vi "UpdateStatus.vi"(8 "error in (no error)":errorcluster, 10 "status":string, 11 "Interface in":refnum<class "Interface.lvclass">) -> (0 "error out":errorcluster, 3 "Interface out":refnum<class "Interface.lvclass">)   [LabVIEW 2018, in "Interface.lvclass"]
uses:
  Interface.lvclass
  Interface.lvclass/Interface.ctl
panel:
  in  "Camera Status":T1
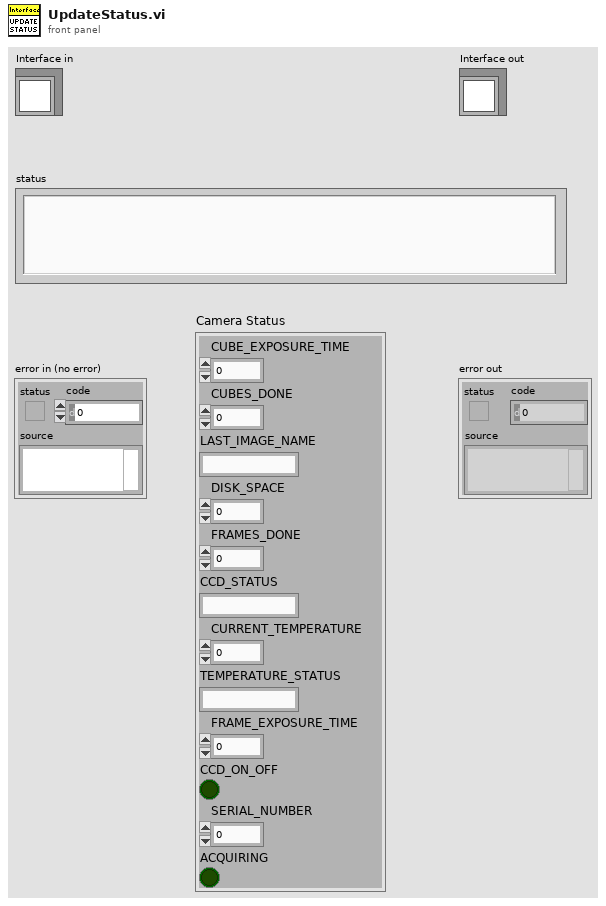
[diagram p1: front panel]
types:
  T1 = cluster{"CUBE_EXPOSURE_TIME":sgl, "CUBES_DONE":u16, "LAST_IMAGE_NAME":string, "DISK_SPACE":u16, "FRAMES_DONE":u16, "CCD_STATUS":string, "CURRENT_TEMPERATURE":i16, "TEMPERATURE_STATUS":string, "FRAME_EXPOSURE_TIME":u16, "CCD_ON_OFF":bool, "SERIAL_NUMBER":u16, "ACQUIRING":bool}
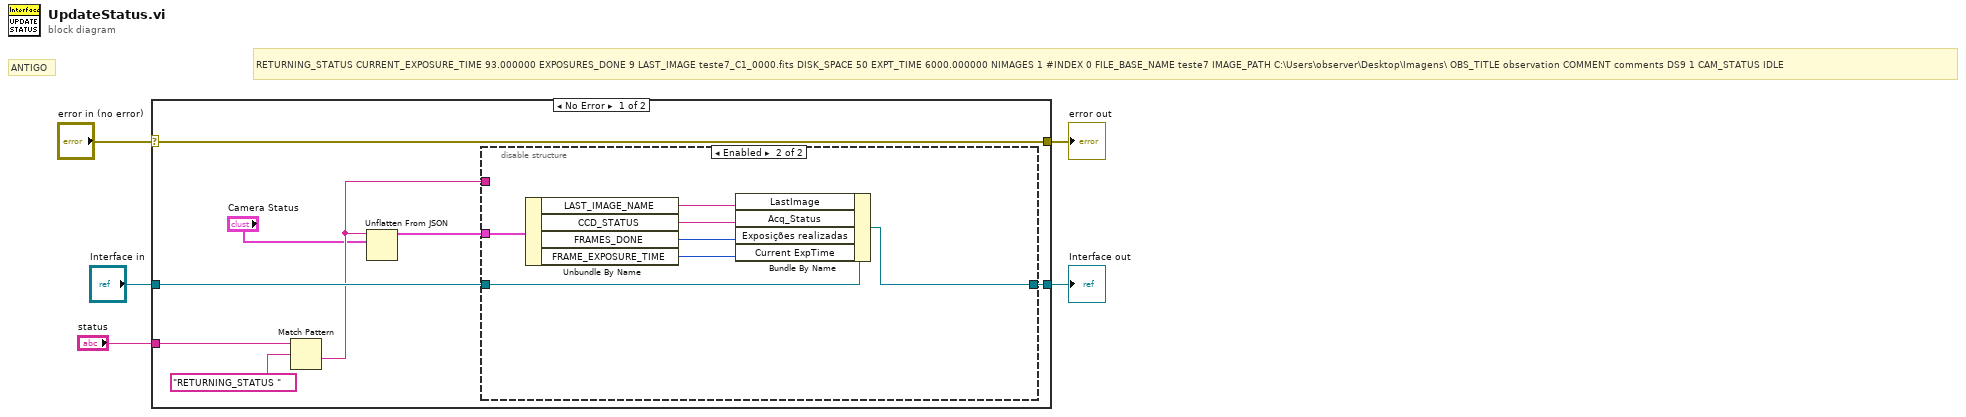
[diagram p0: block diagram]
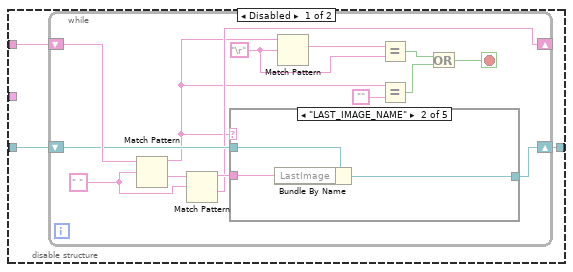
[diagram p2: hidden frame]
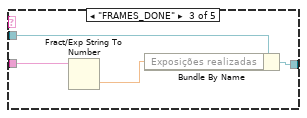
[diagram p4: hidden frame]
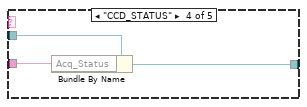
[diagram p5: hidden frame]
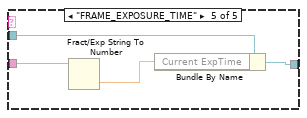
[diagram p6: hidden frame]
diagram:
  # "ANTIGO"
  # "RETURNING_STATUS CURRENT_EXPOSURE_TIME 93.000000 EXPOSURES_DONE 9 LAST_IMAGE teste7_C1_0000.fits DISK_SPACE 50 EXPT_TIME 6000.000000 NIMAGES 1 #INDEX 0 FILE_BASE_NAME teste7 IMAGE_PATH C:\\Users\\observer\\Desktop\\Imagens\\ OBS_TITLE observation COMMENT comments DS9 1 CAM_STATUS IDLE"
  n1 = case shown="No Error" "error in (no error)" {
    selector: "error in (no error)" -> [w13 w54]
    tunnel: [w13 w54] -> w4
    tunnel: [w11 w53] -> w2
    tunnel: "Interface in" -> [w12 w53]
    tunnel: "status" -> [w9 _]
    frame No Error {
      n2 = Match Pattern(string=w9, regular expression="RETURNING_STATUS ") -> (after substring=w8:string)  [unwired: 1 in, 3 out]
      n3 = Unflatten From JSON(JSON string=w8, type and defaults="Camera Status") -> (value=w6:T1)  [unwired: 5 in, 1 out]
      n4 = disable-structure shown="Enabled" {
        disable-tunnel: w12 -> [w16 w51]
        disable-tunnel: [w15 w49] -> w11
        disable-tunnel: w8 -> [w14 _]
        disable-tunnel: w6 -> [_ w52]
        frame Disabled {
          n5 = while {
            shift-right: [w25] -> _
            shift-left: w14 -> [w30]
            shift-right: [w26] -> w15
            shift-left: w16 -> [w27]
            stop <- w20 stop-if-true
            w23 = " "
            w24 = "\r" ("regular expression")
            n6 = Match Pattern(string=w30, regular expression=w23) -> (before substring=w17:string, after substring=w29:string)  [unwired: 1 in, 2 out]
            n7 = Match Pattern(string=w29, regular expression=w23) -> (before substring=w28:string, after substring=w25:string)  [unwired: 1 in, 2 out]
            n8 = case shown="\"LAST_IMAGE_NAME\"" w17 {
              tunnel: w28 -> [_ w32 w35 w39 w43]
              tunnel: w27 -> [w31 w34 w38 w41 w45]
              tunnel: [w31 w33 w37 w40 w44] -> w26
              frame Default {
              }
              frame "LAST_IMAGE_NAME" {
                n9 = Bundle By Name(cluster=w34, "LastImage"=w32) -> (w33:refnum<class "Interface.lvclass">)
              }
              frame "FRAMES_DONE" {
                n10 = Fract/Exp String To Number(string=w35) -> (number=w36:dbl)  [unwired: 3 in, 1 out]
                n11 = Bundle By Name(cluster=w38, "Exposições realizadas"=w36) -> (w37:refnum<class "Interface.lvclass">)
              }
              frame "CCD_STATUS" {
                n12 = Bundle By Name(cluster=w41, "Acq_Status"=w39) -> (w40:refnum<class "Interface.lvclass">)
              }
              frame "FRAME_EXPOSURE_TIME" {
                n13 = Fract/Exp String To Number(string=w43) -> (number=w42:dbl)  [unwired: 3 in, 1 out]
                n14 = Bundle By Name(cluster=w45, "Current ExpTime"=w42) -> (w44:refnum<class "Interface.lvclass">)
              }
            }
            n15 = Match Pattern(string=w17, regular expression=w24) -> (match substring=w19:string)  [unwired: 1 in, 3 out]
            n16 = Equal?(x=w19, y=w24) -> (x = y?=w22:bool)
            n17 = Equal?(x=w17, y="") -> (x = y?=w21:bool)
            n18 = Or(x=w22, y=w21) -> (x .or. y?=w20:bool)
          }
        }
        frame Enabled {
          n19 = Unbundle By Name(w52) -> ("LAST_IMAGE_NAME"=w46:string, "CCD_STATUS"=w47:string, "FRAMES_DONE"=w48:u16, "FRAME_EXPOSURE_TIME"=w50:u16)
          n20 = Bundle By Name(cluster=w51, "LastImage"=w46, "Acq_Status"=w47, "Exposições realizadas"=w48, "Current ExpTime"=w50) -> (w49:refnum<class "Interface.lvclass">)
        }
      }
    }
    frame Error {
    }
  }
  "error out" <- w4
  "Interface out" <- w2
